vi "Main.vi"() -> ()   [LabVIEW 2017, in "TemplatePatternDemo.lvclass"]
uses:
  TemplatePatternDemo.lvclass
  ConsoleOut/Print Options.ctl
  Game Class/Game.lvclass
  Cricket Class/Cricket.lvclass
  C:/Users/fflores/Documents/LabVIEW-Open-Projects/LabIVEW OOP Design Patterns/Template Pattern/Game Class/Game.lvclass
  Football Class/Football.lvclass
panel:
  in  "Game Selector":enum16{"<Select a Game>", "Cricket", "Football"}(ring)
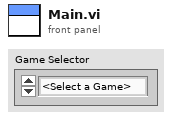
[diagram p1: front panel]
types:
  T1 = typedef "Print Options.ctl" = enum16{"Create", "Get Reference", "Print", "Print Header", "Close"}
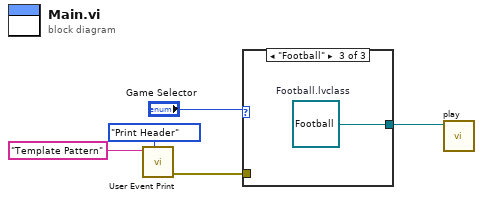
[diagram p0: block diagram]
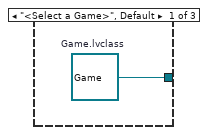
[diagram p2: hidden frame]
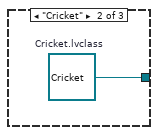
[diagram p3: hidden frame]
diagram:
  n1 = call "User Event Print.vi"("Options"=Print_Options."Print Header", "String to Print"="Template Pattern") -> ("error out"=w3:errorcluster)  [unwired: 8 in, 1 out]
  n2 = case shown="\"Football\"" "Game Selector" {
    tunnel: [w6 w7 w8] -> w4
    tunnel: w3 -> [_ _ _]
    frame "<Select a Game>", Default {
      w6 = refnum<class "Game.lvclass"> refnum  # Game.lvclass
    }
    frame "Cricket" {
      w7 = refnum<class "Cricket.lvclass"> refnum  # Cricket.lvclass
    }
    frame "Football" {
      w8 = refnum<class "Football.lvclass"> refnum  # Football.lvclass
    }
  }
  n3 = call "play.vi"("Game in"=w4) -> ()  [unwired: 9 in, 2 out]
